vi "Web DAV Namen cRio Daten.vi"(7 "IP Adresse":string, 8 "error in":errorcluster, 11 "startup":bool) -> (0 "error out":errorcluster, 2 "Pfad cRio":string, 3 "Dateien FTP":string[](array[string]))   [LabVIEW 2020, in "Backup.lvlib"]
uses:
  Backup.lvlib
  <vilib>/FTP/NI_FTP.lvlib
  <vilib>/WebDAVClient/NI_WebDAV.lvlib
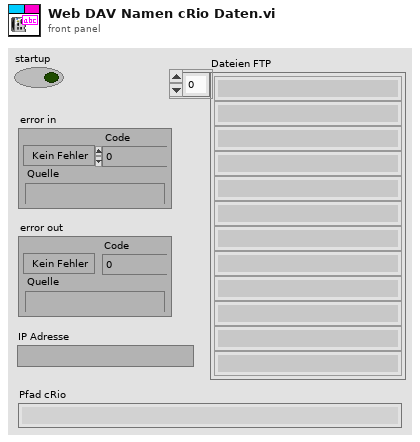
[diagram p1: front panel]
types:
  T1 = typedef "NI_FTP.lvlib/FTP Session.ctl" = refnum<k5>
  T2 = typedef "NI_FTP.lvlib/FTP File Info.ctl" = cluster{"type":enum16{"unknown", "file", "dir", "link"}, "permissions":string, "owner":string, "group":string, "size":i32, "date":string, "name":string, "link name":string}
  T3 = typedef "NI_WebDAV.lvlib/SessionHandle.ctl" = refnum<k1>
  T4 = typedef "NI_WebDAV.lvlib/FileInfo.ctl" = cluster{"type":string, "size":u64, "last modification":timestamp, "display name":string, "uri":string}
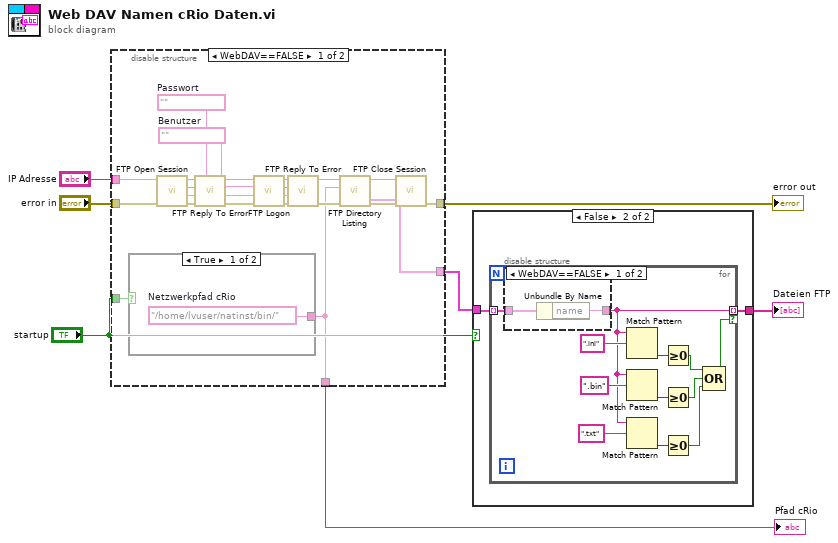
[diagram p0: block diagram]
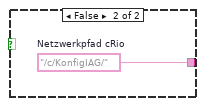
[diagram p2: hidden frame]
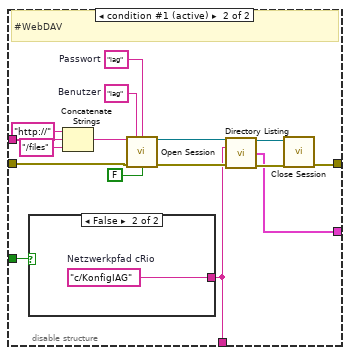
[diagram p3: hidden frame]
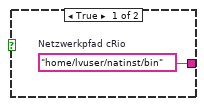
[diagram p4: hidden frame]
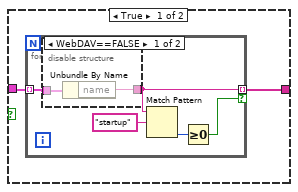
[diagram p5: hidden frame]
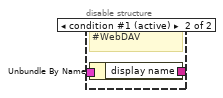
[diagram p6: hidden frame]
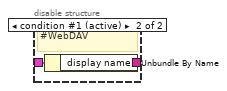
[diagram p7: hidden frame]
diagram:
  n1 = disable-structure shown="WebDAV==FALSE" {
    disable-tunnel: [w29 w32] -> w6
    disable-tunnel: [w8 w36] -> w5
    disable-tunnel: "error in" -> [w14 w44]
    disable-tunnel: [w13 w33] -> w3
    disable-tunnel: "IP Adresse" -> [w12 w45]
    disable-tunnel: "startup" -> [w9 w37]
    frame condition #0 {
      w11 = ""  # Passwort
      w10 = ""  # Benutzer
      n2 = case shown="True" w9 {
        tunnel: [w30 w31] -> w8
        frame True {
          w30 = "/home/lvuser/natinst/bin/"  # Netzwerkpfad cRio
        }
        frame False {
          w31 = "/c/KonfigIAG/"  # Netzwerkpfad cRio
        }
      }
      n3 = call <vilib>:"FTP Open Session.vi"("error in (no error)"=w14, "address"=w12) -> ("error out"=w19:errorcluster, "reply string"=w18:string, "reply code"=w17:i32, "ftp session"=w16:T1)  [unwired: 6 in]
      n4 = call <vilib>:"FTP Reply To Error.vi"("error in (no error)"=w19, "reply string in"=w18, "reply code in"=w17, "ftp session"=w16) -> ("error out"=w20:errorcluster, "ftp session out"=w15:T1)  [unwired: 2 out]
      n5 = call <vilib>:"FTP Logon.vi"("error in (no error)"=w20, "password"=w11, "user"=w10, "ftp session"=w15) -> ("error out"=w24:errorcluster, "reply string"=w23:string, "reply code"=w22:i32, "ftp session out"=w21:T1)  [unwired: 4 in]
      n6 = call <vilib>:"FTP Reply To Error.vi"("error in (no error)"=w24, "reply string in"=w23, "reply code in"=w22, "ftp session"=w21) -> ("error out"=w25:errorcluster, "ftp session out"=w26:T1)  [unwired: 2 out]
      n7 = call <vilib>:"FTP Directory Listing.vi"("error in (no error)"=w25, "directory path"=w8, "ftp session"=w26) -> ("error out"=w27:errorcluster, "ftp session out"=w28:T1, "dir list"=w29:T2[])  [unwired: 4 in, 2 out]
      n8 = call <vilib>:"FTP Close Session.vi"("error in (no error)"=w27, "ftp session"=w28) -> ("error out"=w13:errorcluster)  [unwired: 6 in, 3 out]
    }
    frame condition #1 (active) {
      w42 = "iag"  # Passwort
      w41 = "iag"  # Benutzer
      # "#WebDAV"
      n9 = case shown="False" w37 {
        tunnel: [w48 w49] -> w36
        frame True {
          w48 = "home/lvuser/natinst/bin"  # Netzwerkpfad cRio
        }
        frame False {
          w49 = "c/KonfigIAG"  # Netzwerkpfad cRio
        }
      }
      n10 = Concatenate Strings("http://" ("String"), w45, "/files" ("String")) -> (w40:string)
      n11 = call <vilib>:"Open Session.vi"("host uri prefix"=w40, "username"=w41, "password"=w42, "error in (no error)"=w44, "verify server?"=FALSE) -> ("session handle out"=w46:T3, "error out"=w47:errorcluster)  [unwired: 9 in]
      n12 = call <vilib>:"Directory Listing.vi"("session handle"=w46, "relative uri"=w36, "error in (no error)"=w47) -> ("session handle out"=w35:T3, "file list"=w32:T4[], "error out"=w34:errorcluster)  [unwired: 9 in, 1 out]
      n13 = call <vilib>:"Close Session.vi"("session handle"=w35, "error in (no error)"=w34) -> ("error out"=w33:errorcluster)  [unwired: 13 in]
    }
  }
  "error out" <- w3
  "Pfad cRio" <- w5
  n14 = case shown="False" "startup" {
    tunnel: w6 -> [w51 w62]
    tunnel: [w50 w61] -> w7
    frame True {
      n15 = for {
        tunnel: w51 -> [w56] mode=indexing
        tunnel: [w55] -> w50 mode=indexing if=w53
        n16 = disable-structure shown="WebDAV==FALSE" {
          disable-tunnel: w56 -> [w58 w60]
          disable-tunnel: [w57 w59] -> w55
          frame condition #0 {
            n17 = Unbundle By Name(w58) -> ("name"=w57:string)
          }
          frame condition #1 (active) {
            # "#WebDAV"
            n18 = Unbundle By Name(w60) -> ("display name"=w59:string)
          }
        }
        n19 = Match Pattern(string=w55, regular expression="startup" ("Regulärer Ausdruck")) -> (offset past match=w54:i32)  [unwired: 1 in, 3 out]
        n20 = Greater Or Equal To 0?(x=w54) -> (x >= 0?=w53:bool)
      }
    }
    frame False {
      n21 = for {
        tunnel: w62 -> [w74] mode=indexing
        tunnel: [w65] -> w61 mode=indexing if=w67
        n22 = disable-structure shown="WebDAV==FALSE" {
          disable-tunnel: w74 -> [w76 w78]
          disable-tunnel: [w75 w77] -> w65
          frame condition #0 {
            n23 = Unbundle By Name(w76) -> ("name"=w75:string)
          }
          frame condition #1 (active) {
            # "#WebDAV"
            n24 = Unbundle By Name(w78) -> ("display name"=w77:string)
          }
        }
        n25 = Match Pattern(string=w65, regular expression=".ini" ("Regulärer Ausdruck")) -> (offset past match=w73:i32)  [unwired: 1 in, 3 out]
        n26 = Match Pattern(string=w65, regular expression=".bin" ("Regulärer Ausdruck")) -> (offset past match=w71:i32)  [unwired: 1 in, 3 out]
        n27 = Match Pattern(string=w65, regular expression=".txt" ("Regulärer Ausdruck")) -> (offset past match=w64:i32)  [unwired: 1 in, 3 out]
        n28 = Greater Or Equal To 0?(x=w73) -> (x >= 0?=w68:bool)
        n29 = Greater Or Equal To 0?(x=w71) -> (x >= 0?=w69:bool)
        n30 = Greater Or Equal To 0?(x=w64) -> (x >= 0?=w63:bool)
        n31 = Compound Arithmetic op=OR ("Mehrfacharithmetik")(w68, w69, w63) -> (w67:bool)
      }
    }
  }
  "Dateien FTP" <- w7
